vi "BasePixelCalib.vi"(8 "error in (no error)":errorcluster, 11 "MagSpec_Bella in":refnum<class "MagSpec_Bella.lvclass">) -> (0 "error out":errorcluster, 3 "MagSpec_Bella out":refnum<class "MagSpec_Bella.lvclass">)   [LabVIEW 2020, in "MagSpec_Bella.lvclass"]
uses:
  MagSpec_Bella.lvclass
  MagSpec_Bella.lvclass/MagSpec_Bella.ctl
  OnOffTypeDef.ctl
  NI_AALPro.lvlib
  NI_AALBase.lvlib
panel:
  out "XY Graph":cluster{dbl[], "Array out":dbl[]}[](graph)
  out "bending angle Side":dbl[](graph)
  out "bending angle Front":dbl[](graph)
  out "energy dependence":dbl[][](graph)
  out "bending angle":dbl[][](graph)
  out "pixel angle":dbl[][](graph)
  out "position":dbl[][](graph)
  out "Array":dbl[](array[numeric])
  out "total path":dbl[][](graph)
  out "dp/B":dbl[][](graph)
  out "Width":dbl[](array[numeric])
  out "index":dbl[](array[numeric])
  out "index":dbl[][](graph)
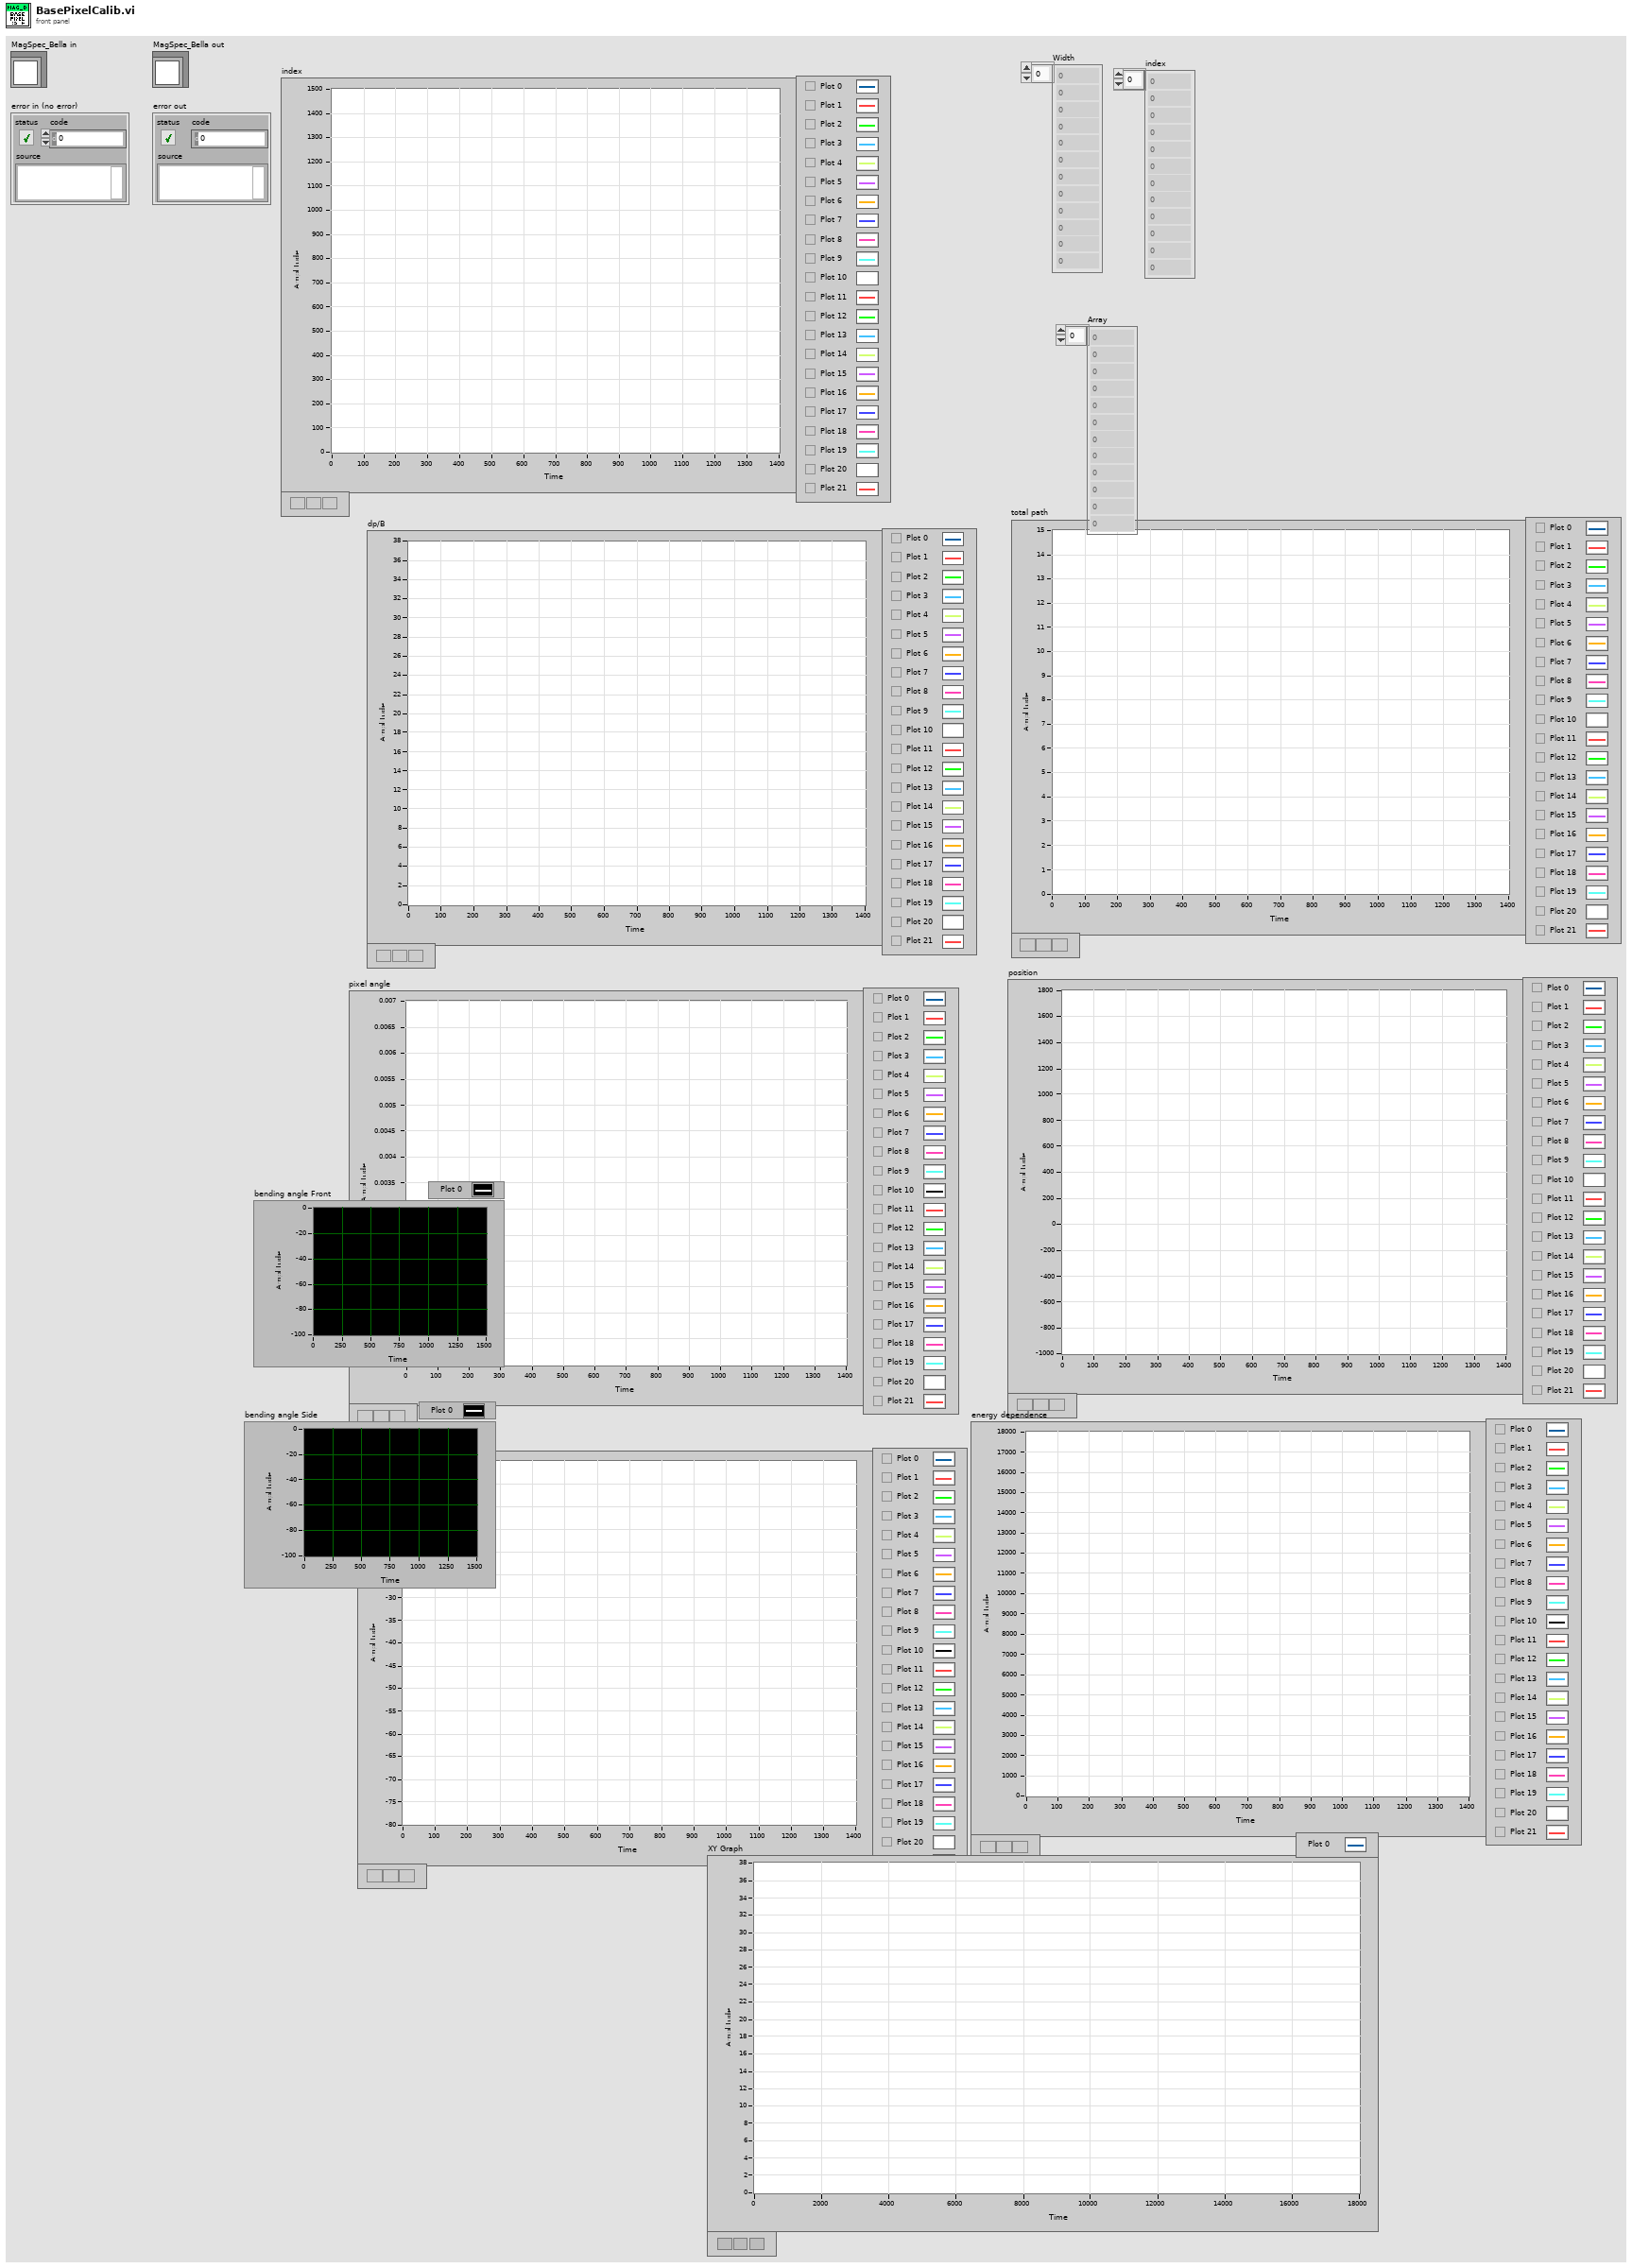
[diagram p1: front panel]
types:
  T1 = typedef "CameraSettings_File.ctl" = cluster{"FOV [mm]":dbl, "Left edge [mm]":dbl, "ROI Y offset":dbl, "ROI height":dbl, "ROI X offset":dbl, "ROI width":dbl, "Y center pixel":dbl, "Y Start":dbl, "Y End":dbl, "X Start":dbl, "X End":dbl, "rot [deg]":dbl}
  T2 = typedef "Calibration_Pixel_based.ctl" = cluster{"y1(pixel)":dbl[], "y2(pixel)":dbl[], "dp/B [MeV/C/B] (pixel)":dbl[], "energyDependence Input(pixel)":dbl[], "bending angle [deg](pixel)":dbl[], "total path(pixel)":dbl[], "pixel angle (y)(pixel)":dbl[], "energy dependence (pixel)":dbl[], "charge compensation (pixel)":dbl[], "Momentum [MeV/C](pixel)":dbl[], "angular compensation(pixel)":dbl[]}
  T3 = typedef "CalibrationCluster.ctl" = cluster{"bending angle Front":dbl[], "bending angle Side":dbl[], "screen [m] Front":dbl[], "screen [m] Side":dbl[], "momentum [MeV/c]":dbl[], "total path [m]":dbl[], "x[mm](rms)":dbl[], "x[mm](rms,b)":dbl[], "y[mm](rms)":dbl[], "y[mm](rms,b)":dbl[]}
  T4 = typedef "OneTimeCalculation.ctl" = cluster{"first Pixel pos [m]":dbl, "Pixel Size [mm]":dbl, "forward":T5}
  T5 = typedef "OnOffTypeDef.ctl" = enum16{"off", "on"}
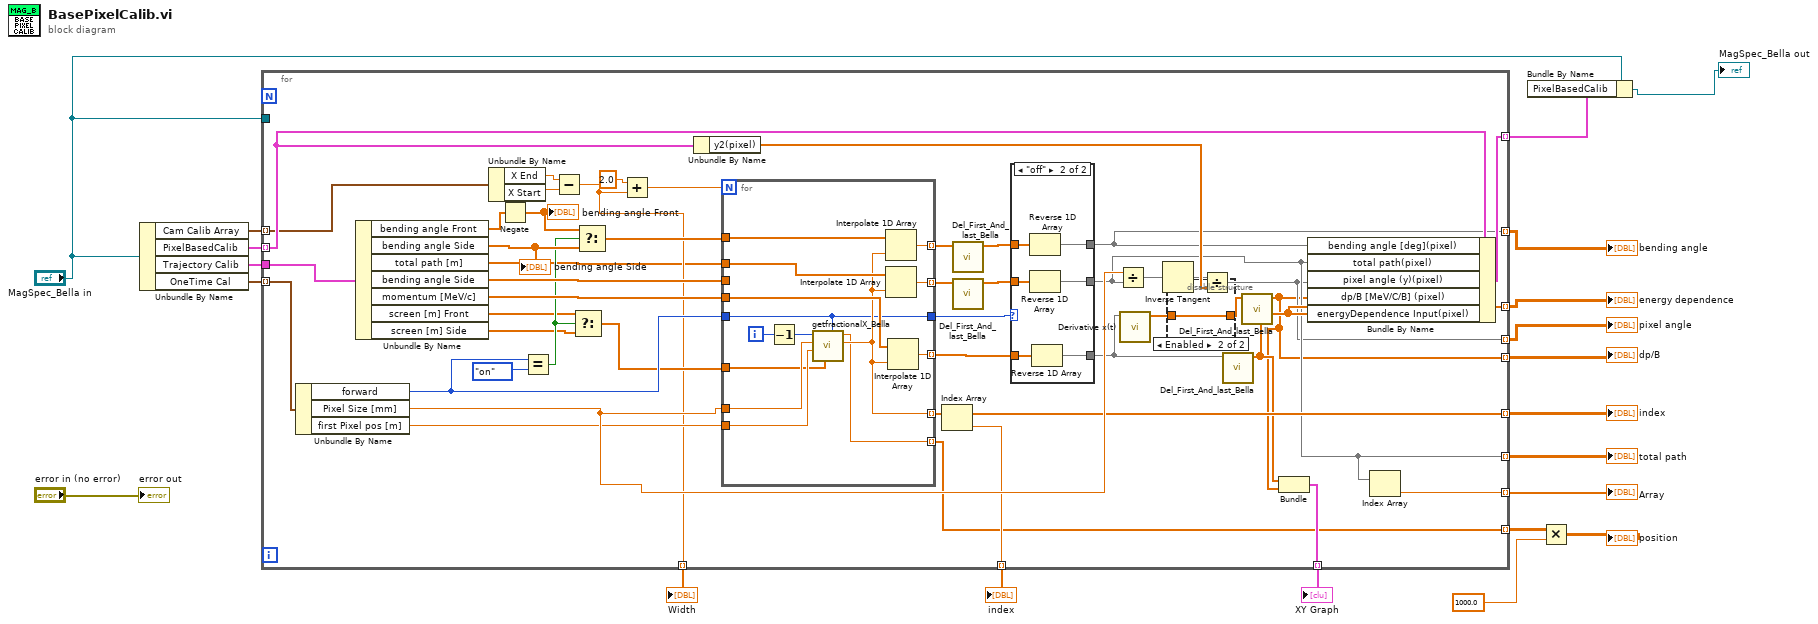
[diagram p0: block diagram]
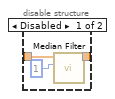
[diagram p2: hidden frame]
diagram:
  n1 = Unbundle By Name("MagSpec_Bella in") -> ("Cam Calib Array"=w13:T1[], "PixelBasedCalib"=w17:T2[], "Trajectory Calib"=w15:T3, "OneTime Cal"=w16:T4[])
  n2 = for {
    tunnel: "MagSpec_Bella in" -> [_]
    tunnel: w15 -> [w56]
    tunnel: w16 -> [w55] mode=indexing
    tunnel: w17 -> [w53] mode=indexing
    tunnel: [w52] -> w18 mode=indexing
    tunnel: [w40] -> w14 mode=indexing
    tunnel: w13 -> [w45] mode=indexing
    tunnel: [w41] -> w12 mode=indexing
    tunnel: [w34] -> w11 mode=indexing
    tunnel: [w22] -> w10 mode=indexing
    tunnel: [w24] -> w9 mode=indexing
    tunnel: [w32] -> w8 mode=indexing
    tunnel: [w28] -> w7 mode=indexing
    tunnel: [w23] -> w4 mode=indexing
    tunnel: [w26] -> w3 mode=indexing
    tunnel: [w27] -> w2 mode=indexing
    tunnel: [w29] -> w1 mode=indexing
    n3 = Unbundle By Name(w55) -> ("forward"=w44:T5, "Pixel Size [mm]"=w67:dbl, "first Pixel pos [m]"=w54:dbl)
    n4 = Unbundle By Name(w56) -> ("bending angle Front"=w30:dbl[], "bending angle Side"=w51:dbl[], "total path [m]"=w33:dbl[], "bending angle Side"=w46:dbl[], "momentum [MeV/c]"=w47:dbl[], "screen [m] Front"=w37:dbl[], "screen [m] Side"=w38:dbl[])
    "bending angle Side" <- w51
    n5 = Unbundle By Name(w45) -> ("X End"=w36:dbl, "X Start"=w35:dbl)
    n6 = Negate(x=w30) -> (-x=w25:dbl[])
    "bending angle Front" <- w25
    n7 = Equal?(x=w44, y=OnOffTypeDef."on") -> (x = y?=w43:bool)
    n8 = Subtract(x=w36, y=w35) -> (x-y=w34:dbl)
    n9 = Select(t=w37, s=w43, f=w38) -> (s? t:f=w42:dbl[])
    n10 = Select(t=w25, s=w43, f=w51) -> (s? t:f=w50:dbl[])
    n11 = Add(x=2.0, y=w34) -> (x+y=w39:dbl)
    n12 = Unbundle By Name(w53) -> ("y2(pixel)"=w68:dbl[])
    n13 = for {
      N: w39 -> [_]
      tunnel: w67 -> [w95]
      tunnel: w54 -> [w94]
      tunnel: w50 -> [w93]
      tunnel: w46 -> [_]
      tunnel: [w92] -> w60 mode=indexing
      tunnel: w47 -> [w91]
      tunnel: [w90] -> w57 mode=indexing
      tunnel: w33 -> [w86]
      tunnel: [w89] -> w65 mode=indexing
      tunnel: w44 -> [w83]
      tunnel: [w83] -> w31
      tunnel: [w85] -> w40 mode=indexing
      tunnel: w42 -> [w84]
      tunnel: [w82] -> w28 mode=indexing
      i -> [w88]
      n14 = Decrement(x=w88) -> (x-1=w87:i32)
      n15 = call "getfractionalX_Bella.vi"("CameraFlipped"=w83, "screen [m]"=w84, "position [m]"=w94, "pixelsize"=w95, "position index"=w87) -> ("index"=w85:dbl, "position m"=w82:dbl)  [unwired: 5 in]
      n16 = Interpolate 1D Array(1:w85, 2:w93) -> (0:w92:dbl)
      n17 = Interpolate 1D Array(1:w85, 2:w86) -> (0:w89:dbl)
      n18 = Interpolate 1D Array(1:w85, 2:w91) -> (0:w90:dbl)
    }
    n19 = Index Array(array=w40) -> (element=w41:dbl)  [unwired: 1 in]
    n20 = call "Del_First_And_last_Bella.vi"("Array in"=w60) -> ("Array out"=w61:dbl[])  [unwired: 10 in]
    n21 = call "Del_First_And_last_Bella.vi"("Array in"=w65) -> ("Array out"=w66:dbl[])  [unwired: 10 in]
    n22 = case shown="\"off\"" w31 {
      tunnel: w66 -> [w74 w81]
      tunnel: [w75 w80] -> w26
      tunnel: [w74 w79] -> w24
      tunnel: w61 -> [w75 w78]
      tunnel: [w73 w77] -> w48
      tunnel: w57 -> [w73 w76]
      frame "on" {
      }
      frame "off" {
        n23 = Reverse 1D Array(array=w78) -> (reversed array=w80:dbl[])
        n24 = Reverse 1D Array(array=w81) -> (reversed array=w79:dbl[])
        n25 = Reverse 1D Array(array=w76) -> (reversed array=w77:dbl[])
      }
    }
    n26 = Divide(x=w67, y=w24) -> (x/y=w58:dbl[])
    n27 = call "Derivative x(t).vi"("X"=w48) -> ("dX/dt"=w63:dbl[])  [unwired: 9 in, 1 out]
    n28 = Inverse Tangent(1:w58) -> (0:w59:dbl[])
    n29 = disable-structure shown="Enabled" {
      disable-tunnel: [w71 w72] -> w64
      disable-tunnel: w63 -> [w70 w72]
      frame Disabled {
        n30 = call "Median Filter.vi"("left rank"=1, "X"=w70) -> ("Filtered X"=w71:dbl[])  [unwired: 8 in, 1 out]
      }
      frame Enabled {
      }
    }
    n31 = Divide(x=w59, y=w68) -> (x/y=w23:dbl[])
    n32 = call "Del_First_And_last_Bella.vi"("Array in"=w48) -> ("Array out"=w27:dbl[])  [unwired: 10 in]
    n33 = call "Del_First_And_last_Bella.vi"("Array in"=w64) -> ("Array out"=w22:dbl[])  [unwired: 10 in]
    n34 = Bundle("Array out"=w27, "Array out"=w22) -> (w29:cluster{"Array out":dbl[], "Array out":dbl[]})  [unwired: 1 in]
    n35 = Bundle By Name(cluster=w53, "bending angle [deg](pixel)"=w26, "total path(pixel)"=w24, "pixel angle (y)(pixel)"=w23, "dp/B [MeV/C/B] (pixel)"=w22, "energyDependence Input(pixel)"=w27) -> (w52:T2)
    n36 = Index Array(array=w24) -> (element=w32:dbl)  [unwired: 1 in]
  }
  "index" <- w14
  "index" <- w12
  "Width" <- w11
  "dp/B" <- w10
  "total path" <- w9
  "Array" <- w8
  "pixel angle" <- w4
  "bending angle" <- w3
  "energy dependence" <- w2
  "XY Graph" <- w1
  n37 = Bundle By Name(cluster="MagSpec_Bella in", "PixelBasedCalib"=w18) -> (→"MagSpec_Bella out":refnum<class "MagSpec_Bella.lvclass">)
  n38 = Multiply(x=w7, y=1000.0) -> (x*y=→"position":dbl[][])
  "error out" <- "error in (no error)"
